vi "trio_move_test.vi"() -> ()   [LabVIEW 2017]
uses:
  <instrlib>/Trio Motion/Trio Motion Library.lvlib
panel:
  out "Home status":T1
  in  "Timeout (ms)":u32
  out "Motion error":dbl[](array[numeric])
  out "Move error":errorcluster
  in  "Command":dbl[](array[numeric])=[0.0, 0.0, 0.0, 0.0]
  in  "Axis enable":bool[](array[boolean])=[TRUE, TRUE, TRUE, TRUE]
  in  "Absolute":bool=TRUE
  in  "Do move":bool
  in  "stop":bool
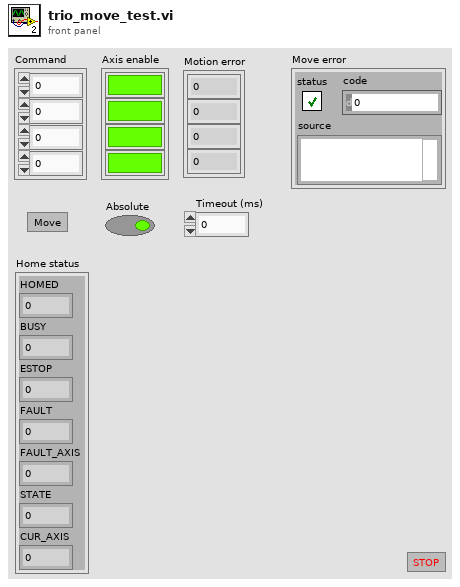
[diagram p1: front panel]
types:
  T1 = cluster{"HOMED":dbl, "BUSY":dbl, "ESTOP":dbl, "FAULT":dbl, "FAULT_AXIS":dbl, "STATE":dbl, "CUR_AXIS":dbl}
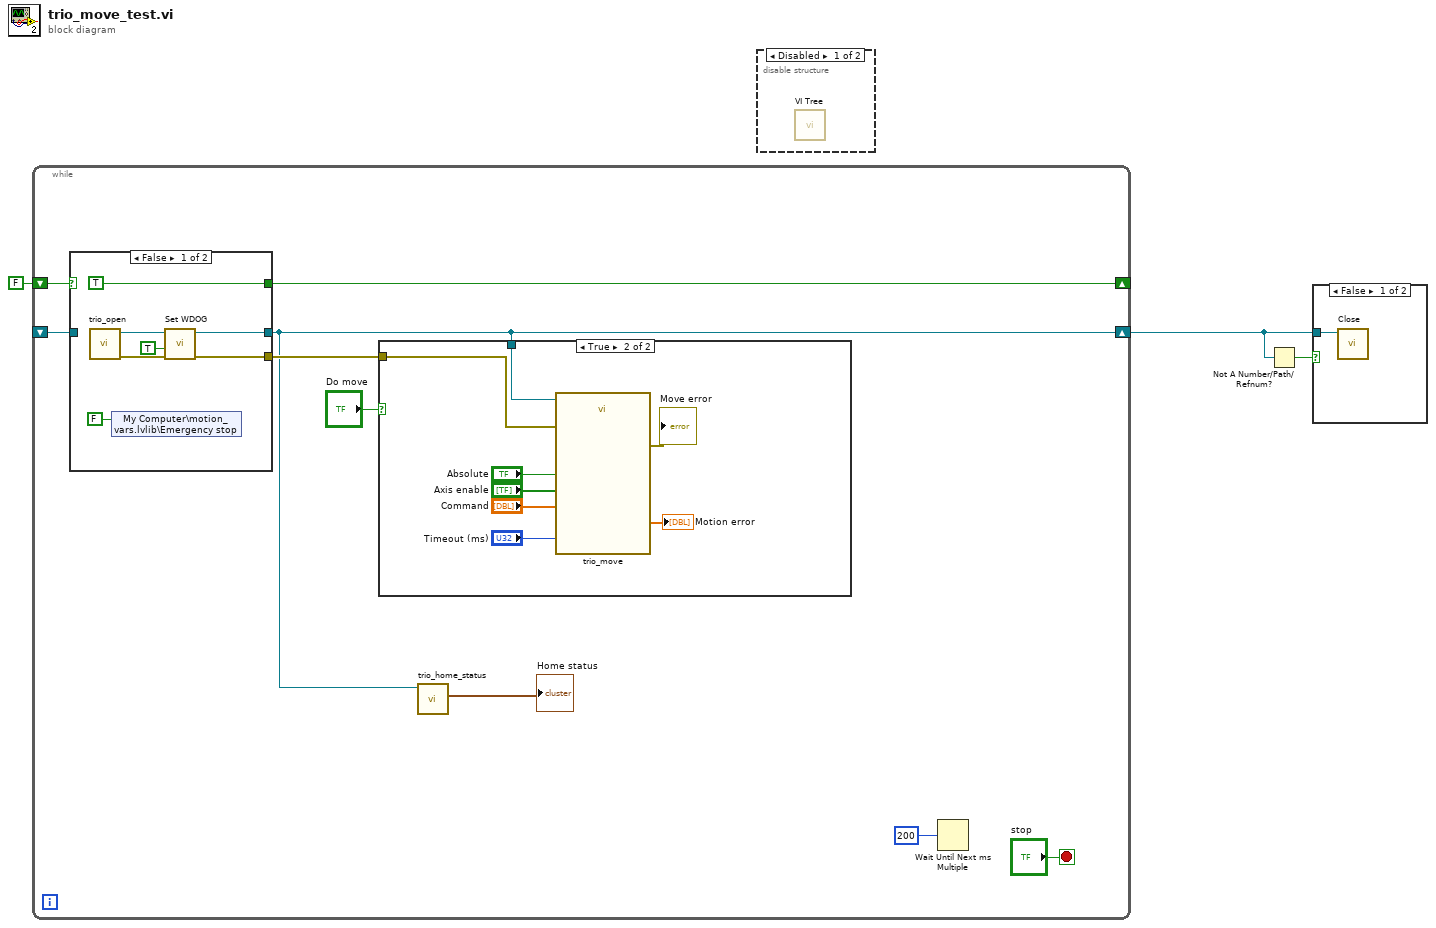
[diagram p0: block diagram]
diagram:
  n1 = while {
    shift-right: [w10] -> _
    shift-left: FALSE -> [w11]
    shift-right: [w5] -> w3
    shift-left: _ -> [w9]
    stop <- "stop" stop-if-true
    n2 = case shown="False" w11 {
      selector: w11 -> [_ w28]
      tunnel: [TRUE w28] -> w10
      tunnel: [w22 w29] -> w5
      tunnel: w9 -> [_ w29]
      tunnel: [w23 _] -> w6
      frame False {
        n3 = call "trio_open.vi"() -> ("error out"=w25:errorcluster, "reference out"=w24:refnum<k7>)  [unwired: 10 in]
        n4 = shared-variable "My Computer\\motion_vars.lvlib\\Emergency stop"(FALSE ("Emergency stop")) -> ()  [unwired: 1 in, 1 out]
        n5 = call <instrlib>:"Set WDOG.vi"("error in (no error)"=w25, "WDOG (ON)"=TRUE, "reference in"=w24) -> ("error out"=w23:errorcluster, "reference out"=w22:refnum<k7>)  [unwired: 6 in, 1 out]
      }
      frame True {
      }
    }
    n6 = case shown="True" "Do move" {
      tunnel: w5 -> [_ w20]
      tunnel: w6 -> [_ w16]
      frame False {
      }
      frame True {
        n7 = call "trio_move.vi"("Axis enable"="Axis enable", "Timeout (ms)"="Timeout (ms)", "error in"=w16, "Axis positions"="Command", "Absolute"="Absolute", "Trio handle"=w20) -> ("error out"=→"Move error":errorcluster, "Motion error"=→"Motion error":dbl[])  [unwired: 4 in]
      }
    }
    n8 = call "trio_home_status.vi"("reference in"=w5) -> ("Status"=→"Home status":T1)  [unwired: 8 in, 2 out]
    n9 = Wait Until Next ms Multiple(millisecond multiple=u32 200) -> ()  [unwired: 1 out]
  }
  n10 = disable-structure shown="Disabled" {
    frame Disabled {
      n11 = call <instrlib>:"VI Tree.vi"() -> ()  [unwired: 12 in]
    }
    frame Enabled {
    }
  }
  n12 = Not A Number/Path/Refnum?(number/path/refnum=w3) -> (NaN/Path/Refnum?=w2:bool)
  n13 = case shown="False" w2 {
    tunnel: w3 -> [w30 _]
    frame False {
      n14 = call <instrlib>:"Close.vi"("reference in"=w30) -> ()  [unwired: 10 in, 1 out]
    }
    frame True {
    }
  }
